vi "Filter String, Pass Scientific Notation.vi"(1 "Input String":string) -> (0 "Numeric String":string)   [LabVIEW 2010]
doc: "Remove all characters except: 0-9, plus, minus, decimal point, e, and E."
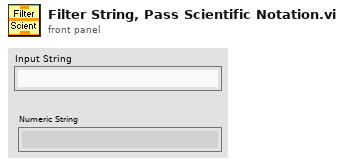
[diagram p1: front panel]
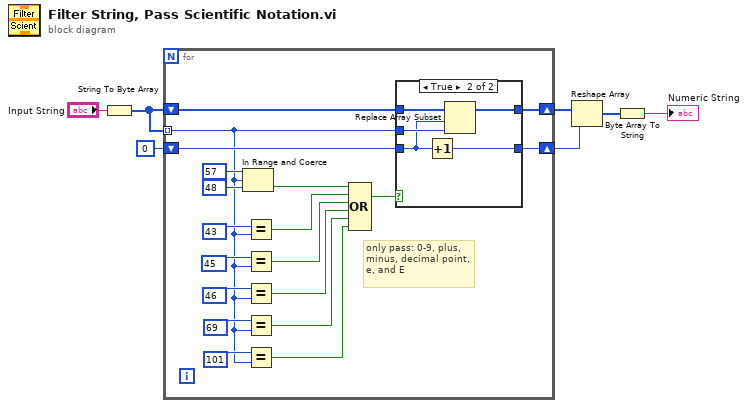
[diagram p0: block diagram]
diagram:
  n1 = String To Byte Array(string="Input String") -> (unsigned byte array=w5:u8[])
  n2 = for {
    tunnel: w5 -> [w8] mode=indexing
    shift-right: [w24] -> w1
    shift-left: 0 ("lower limit") -> [w23]
    shift-right: [w22] -> w4
    shift-left: w5 -> [w21]
    # "only pass: 0-9, plus, minus, decimal point, e, and E"
    n3 = In Range and Coerce(upper limit=u8 57, x=w8, lower limit=u8 48) -> (In Range?=w19:bool)  [unwired: 1 out]
    n4 = Equal?(x=u8 43 ("lower limit"), y=w8) -> (x = y?=w15:bool)
    n5 = Equal?(x=u8 45 ("lower limit"), y=w8) -> (x = y?=w14:bool)
    n6 = Equal?(x=u8 46 ("lower limit"), y=w8) -> (x = y?=w13:bool)
    n7 = Equal?(x=u8 69 ("lower limit"), y=w8) -> (x = y?=w12:bool)
    n8 = Equal?(x=u8 101 ("lower limit"), y=w8) -> (x = y?=w11:bool)
    n9 = Compound Arithmetic op=OR(w19, w15, w14, w13, w12, w11) -> (w20:bool)
    n10 = case shown="True" w20 {
      tunnel: [w28 w33] -> w24
      tunnel: w23 -> [w28 w29]
      tunnel: [w27 w32] -> w22
      tunnel: w21 -> [w27 w31]
      tunnel: w8 -> [_ w30]
      frame False {
      }
      frame True {
        n11 = Increment(x=w29) -> (x+1=w33:i32)
        n12 = Replace Array Subset(array=w31, new element=w30, index=w29) -> (w32:u8[])
      }
    }
  }
  n13 = Reshape Array(w4, w1) -> (w3:u8[])
  n14 = Byte Array To String(unsigned byte array=w3) -> (string=→"Numeric String":string)
